vi "Turn Supply On or Off.vi"(0 "Supply Handle in":refnum<k15>, 1 "Channel Name(s)":string, 5 "Power Mode":T1, 11 "error in (no error)":errorcluster) -> (4 "Supply Handle out":refnum<k15>, 15 "error out":errorcluster)   [LabVIEW 2019, in "Supply.lvlib"]
uses:
  Supply.lvlib
  Typedefs/Supply Power Mode.ctl
  <instrlib>/niDCPower/nidcpower.llb/niDCPower Wait For Event - Event.ctl
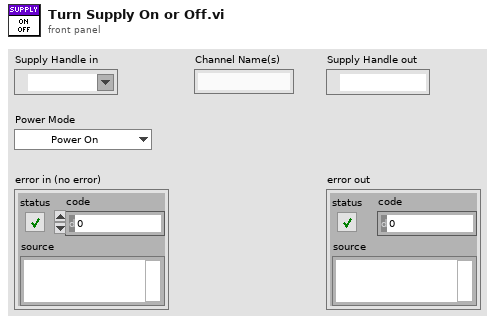
[diagram p1: front panel]
types:
  T1 = typedef "Supply.lvlib/Supply Power Mode.ctl" = enum16{"Power On", "Power Off"}
  T2 = typedef "niDCPower Wait For Event - Event.ctl" = i32
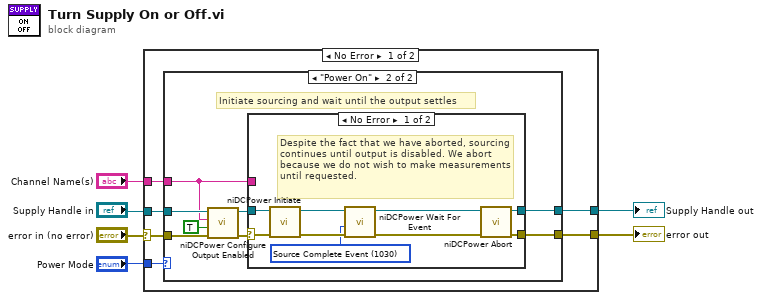
[diagram p0: block diagram]
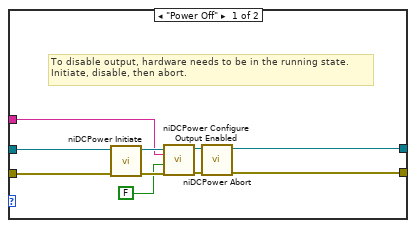
[diagram p2: hidden frame]
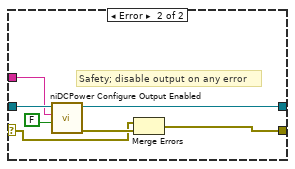
[diagram p3: hidden frame]
diagram:
  n1 = case shown="No Error" "error in (no error)" {
    selector: "error in (no error)" -> [w12 w48]
    tunnel: "Supply Handle in" -> [w11 w47]
    tunnel: "Power Mode" -> [w10 _]
    tunnel: [w9 w48] -> w3
    tunnel: [w8 w47] -> w2
    tunnel: "Channel Name(s)" -> [w7 _]
    frame No Error {
      n2 = case shown="\"Power On\"" w10 {
        tunnel: w12 -> [w22 w30]
        tunnel: w11 -> [w19 w26]
        tunnel: [w17 w29] -> w9
        tunnel: [w15 w28] -> w8
        tunnel: w7 -> [w14 w24]
        frame "Power Off" {
          # "To disable output, hardware needs to be in the running state.\nInitiate, disable, then abort."
          n3 = call <instrlib>:"niDCPower Initiate.vi"("error in (no error)"=w22, "instrument handle"=w19) -> ("error out"=w20:errorcluster, "instrument handle out"=w18:refnum<k15>)  [unwired: 8 in]
          n4 = call <instrlib>:"niDCPower Configure Output Enabled.vi"("error in (no error)"=w20, "output enabled"=FALSE, "channel name"=w14, "instrument handle"=w18) -> ("error out"=w21:errorcluster, "instrument handle out"=w16:refnum<k15>)  [unwired: 6 in]
          n5 = call <instrlib>:"niDCPower Abort.vi"("error in (no error)"=w21, "instrument handle"=w16) -> ("error out"=w17:errorcluster, "instrument handle out"=w15:refnum<k15>)  [unwired: 8 in]
        }
        frame "Power On" {
          # "Initiate sourcing and wait until the output settles"
          n6 = call <instrlib>:"niDCPower Configure Output Enabled.vi"("error in (no error)"=w30, "output enabled"=TRUE, "channel name"=w24, "instrument handle"=w26) -> ("error out"=w27:errorcluster, "instrument handle out"=w25:refnum<k15>)  [unwired: 6 in]
          n7 = case shown="No Error" w27 {
            selector: w27 -> [w34 w41]
            tunnel: w25 -> [w33 w46]
            tunnel: [w32 w42] -> w29
            tunnel: [w31 w44] -> w28
            tunnel: w24 -> [_ w40]
            frame No Error {
              w35 = T2 1030 items=["Source Complete Event"=1030, "Measure Complete Event"=1031, "Sequence Iteration Complete Event"=1032, "Sequence Engine Done Event"=1033, "Pulse Complete Event"=1051, "Ready For Pulse Trigger Event"=1052] ("event")
              # "Despite the fact that we have aborted, sourcing continues until output is disabled. We abort because we do not wish to make measurements until requested."
              n8 = call <instrlib>:"niDCPower Initiate.vi"("error in (no error)"=w34, "instrument handle"=w33) -> ("error out"=w36:errorcluster, "instrument handle out"=w37:refnum<k15>)  [unwired: 8 in]
              n9 = call <instrlib>:"niDCPower Wait For Event.vi"("error in (no error)"=w36, "event"=w35, "instrument handle"=w37) -> ("error out"=w39:errorcluster, "instrument handle out"=w38:refnum<k15>)  [unwired: 7 in]
              n10 = call <instrlib>:"niDCPower Abort.vi"("error in (no error)"=w39, "instrument handle"=w38) -> ("error out"=w32:errorcluster, "instrument handle out"=w31:refnum<k15>)  [unwired: 8 in]
            }
            frame Error {
              # "Safety; disable output on any error"
              n11 = call <instrlib>:"niDCPower Configure Output Enabled.vi"("output enabled"=FALSE, "channel name"=w40, "instrument handle"=w46) -> ("error out"=w43:errorcluster, "instrument handle out"=w44:refnum<k15>)  [unwired: 7 in]
              n12 = Merge Errors(w41, w43) -> (w42:errorcluster)
            }
          }
        }
      }
    }
    frame Error {
    }
  }
  "error out" <- w3
  "Supply Handle out" <- w2
